vi "KeyboardInputEvent.vi"(8 "error in":errorcluster, 11 "KeyBoard cluster":cluster{"KeyCode":u8, "dwFlags":u32}) -> (0 "error out":errorcluster)   [LabVIEW 2015]
uses:
  user32.dll
panel:
  # "dwFlafes\n0 -> Key Down\n2 -> Key Up"
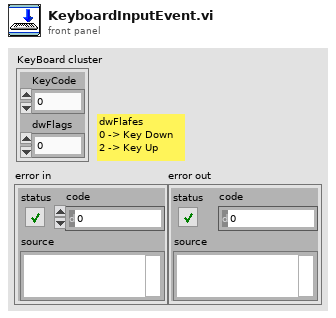
[diagram p1: front panel]
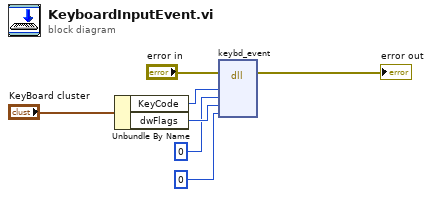
[diagram p0: block diagram]
diagram:
  n1 = Unbundle By Name("KeyBoard cluster") -> ("KeyCode"=w6:u8, "dwFlags"=w5:u32)
  n2 = dll-call lib="user32.dll" fn="keybd_event" label="Call Library Function Node"(error in="error in", "bVk"=w6, "bScan"=u8 0, "dwFlags"=w5, "dwExtraInfo"=u32 0) -> (error out=→"error out":errorcluster)  [unwired: 7 in, 1 out]
